vi "Check Vehicle Position.vi"(8 "error in (no error)":errorcluster, 10 "Right Position":u8=1, 11 "Control Refnum":T1) -> (0 "error out":errorcluster, 3 "Vehicle in position":bool)   [LabVIEW 2024]
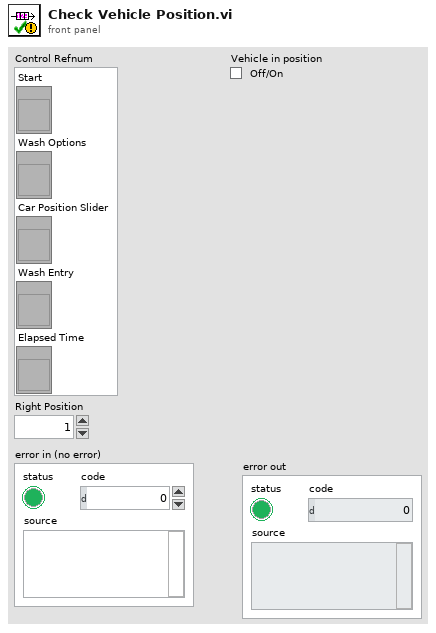
[diagram p1: front panel]
types:
  T1 = cluster{"Start":refnum<vi>, "Wash Options":refnum<vi>, "Car Position Slider":refnum<vi>, "Wash Entry":refnum<vi>, "Elapsed Time":refnum<vi>}
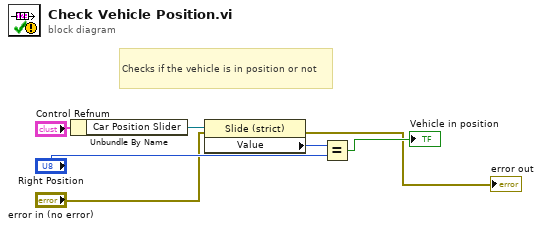
[diagram p0: block diagram]
diagram:
  # "Checks if the vehicle is in position or not"
  n1 = Unbundle By Name("Control Refnum") -> ("Car Position Slider"=w3:refnum<vi>)
  n2 = property class="Slide (strict)"(reference=w3, error in="error in (no error)") -> (error out=→"error out":errorcluster, "Value"=w5:u8)  [unwired: 1 out]
  n3 = Equal?(x=w5, y="Right Position") -> (x = y?=→"Vehicle in position":bool)
